vi "Write Task Updated.vi"(8 "error in (no error)":errorcluster, 10 "Task Updated":refnum<user-event>, 11 "Task Setting Editor in":refnum<class "Task Setting Editor.lvclass">) -> (0 "error out":errorcluster, 3 "Task Setting Editor out":refnum<class "Task Setting Editor.lvclass">)   [LabVIEW 2017, in "Task Setting Editor.lvlib" / "Task Setting Editor.lvclass"]
uses:
  Task Setting Editor.lvclass
  Classes/Task Interface/Task/Task.lvclass
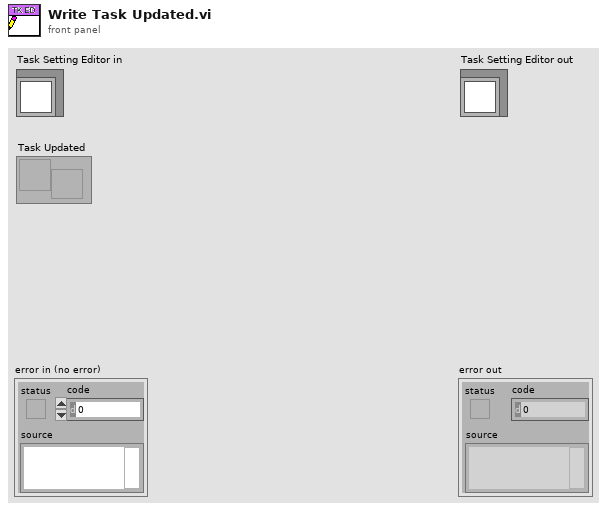
[diagram p1: front panel]
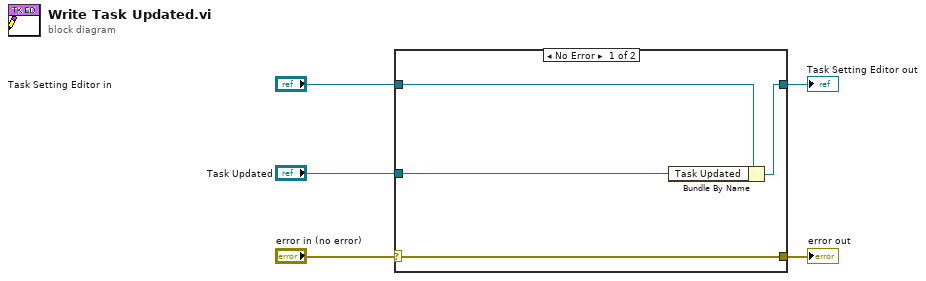
[diagram p0: block diagram]
diagram:
  n1 = case shown="No Error" "error in (no error)" {
    selector: "error in (no error)" -> [w9 w10]
    tunnel: [w9 w10] -> w4
    tunnel: [w7 w11] -> w2
    tunnel: "Task Setting Editor in" -> [w8 w11]
    tunnel: "Task Updated" -> [w6 _]
    frame No Error {
      n2 = Bundle By Name(cluster=w8, "Task Updated"=w6) -> (w7:refnum<class "Task Setting Editor.lvclass">)
    }
    frame Error {
    }
  }
  "error out" <- w4
  "Task Setting Editor out" <- w2
